vi "Laser-On.vi"(2 "error in (no error)":errorcluster, 5 "VISA resource name":refnum<visa-resource-name>) -> (0 "error out":errorcluster, 1 "VISA resource name out":refnum<visa-resource-name>)   [LabVIEW 2013]
panel:
  # "uJ"
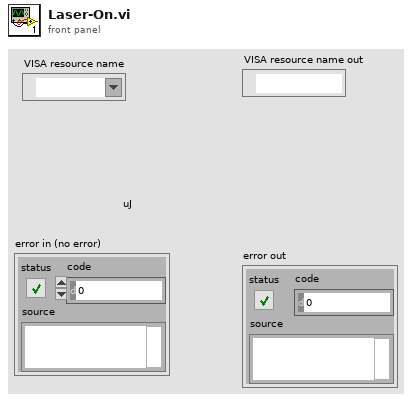
[diagram p1: front panel]
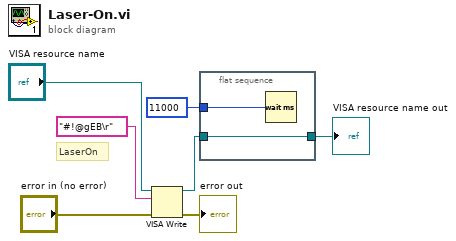
[diagram p0: block diagram]
diagram:
  # "LaserOn"
  n1 = VISA Write(VISA resource name="VISA resource name", write buffer="#!@gEB\r", error in (no error)="error in (no error)") -> (VISA resource name out=w3:refnum<visa-resource-name>, error out=→"error out":errorcluster)  [unwired: 1 out]
  n2 = flat-sequence {
    tunnel: w3 -> [w9]
    tunnel: [w9] -> w2
    tunnel: u32 11000 ("delay before read (ms)") -> [w8]
    frame #0 {
      n3 = Wait (ms)(milliseconds to wait=w8) -> ()  [unwired: 1 out]
    }
  }
  "VISA resource name out" <- w2
